vi "Evaluate Stop Trigger.vi"(8 "error in (no error)":errorcluster, 10 "Stop Trigger Data":dbl[](array[numeric]), 11 "Triggered Log in":refnum<class "Triggered Log.lvclass">) -> (0 "error out":errorcluster, 3 "Triggered Log out":refnum<class "Triggered Log.lvclass">)   [LabVIEW 2012, in "Triggered Log.lvclass"]
doc: "Evaluate the stop trigger if the log is in the Triggered state. Reset the posttrigger countdown so that when the stop trigger occurs it's ready. If the stop trigger occurs, set the log to the posttrigger state and notify any listeners of the state change."
uses:
  Triggered Log.lvclass
  Triggered Log.lvclass/Triggered Log.ctl
  Triggered Log State.ctl
  On Triggered Log State Change.vi
  Engine/Classes/Triggers/Trigger/Finalize.vi
  Engine/Classes/Triggers/Trigger/Trigger.lvclass
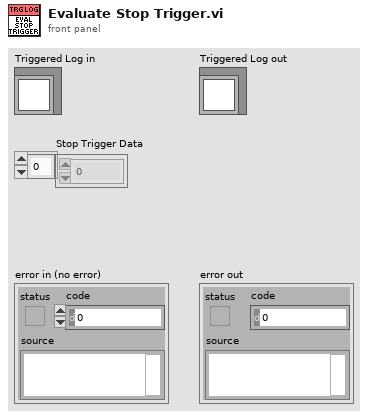
[diagram p1: front panel]
types:
  T1 = typedef "Triggered Log.lvclass/Triggered Log State.ctl" = enum16{"Waiting on Trigger", "Triggered", "Posttrigger", "Complete", "Idle", "Error"}
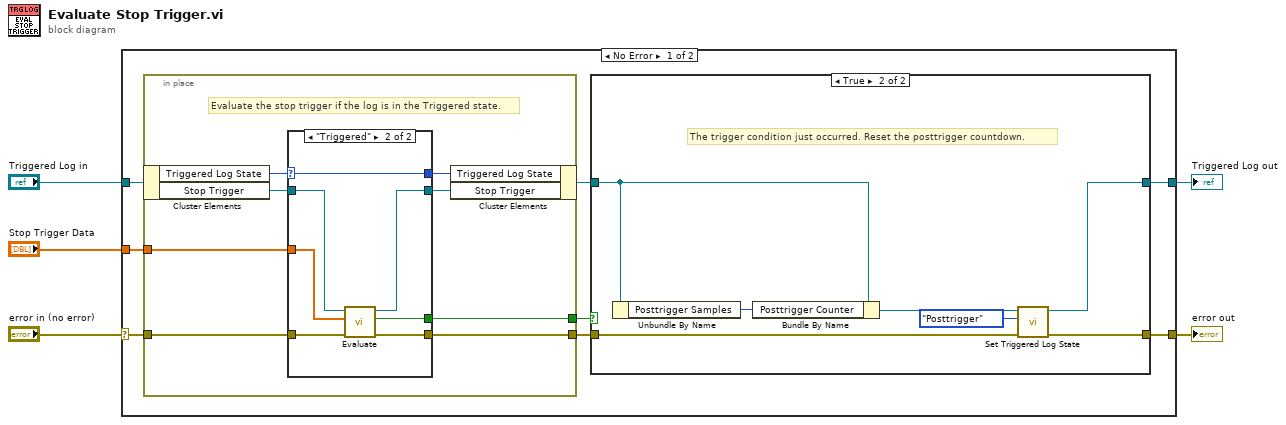
[diagram p0: block diagram]
diagram:
  n1 = case shown="No Error" "error in (no error)" {
    selector: "error in (no error)" -> [w6 w41]
    tunnel: "Stop Trigger Data" -> [w13 _]
    tunnel: "Triggered Log in" -> [w12 w42]
    tunnel: [w9 w41] -> w3
    tunnel: [w8 w42] -> w2
    frame No Error {
      n2 = in-place {
        in-place-border: w6 -> [w21]
        in-place-border: w13 -> [w19]
        in-place-border: [w20] -> w11
        in-place-border: [w16] -> w7
        # "Evaluate the stop trigger if the log is in the Triggered state."
        n3 = in-place-cluster #1(w12) -> ("Triggered Log State"=w17:T1, "Stop Trigger"=w15:refnum<class "Trigger.lvclass">)
        n4 = case shown="\"Triggered\"" w17 {
          selector: w17 -> [w24 w31]
          tunnel: w15 -> [w23 w30]
          tunnel: [w23 w26] -> w14
          tunnel: w21 -> [w22 w29]
          tunnel: [w22 w28] -> w20
          tunnel: w19 -> [_ w27]
          tunnel: [w24 w31] -> w18
          tunnel: [_ w25] -> w16
          frame Default {
            # "Only evaluate the trigger if the log is in theTriggered state."
          }
          frame "Triggered" {
            n5 = call "Evaluate.vi"("error in (no error)"=w29, "Trigger Data"=w27, "Trigger in"=w30) -> ("error out"=w28:errorcluster, "Trigger"=w25:bool, "Trigger out"=w26:refnum<class "Trigger.lvclass">)  [unwired: 6 in]
          }
        }
        n6 = in-place-cluster #1("Triggered Log State"=w18, "Stop Trigger"=w14) -> (w10:refnum<class "Triggered Log.lvclass">)
      }
      n7 = case shown="True" w7 {
        tunnel: w11 -> [w32 w38]
        tunnel: [w33 w39] -> w8
        tunnel: w10 -> [w33 w36]
        tunnel: [w32 w40] -> w9
        frame False {
        }
        frame True {
          # "The trigger condition just occurred. Reset the posttrigger countdown."
          n8 = Unbundle By Name(w36) -> ("Posttrigger Samples"=w34:i64)
          n9 = Bundle By Name(cluster=w36, "Posttrigger Counter"=w34) -> (w35:refnum<class "Triggered Log.lvclass">)
          n10 = call "Set Triggered Log State.vi"("error in (no error)"=w38, "Triggered Log State"=Triggered_Log_State."Posttrigger", "Triggered Log in"=w35) -> ("error out"=w40:errorcluster, "Triggered Log out"=w39:refnum<class "Triggered Log.lvclass">)  [unwired: 7 in]
        }
      }
    }
    frame Error {
    }
  }
  "error out" <- w3
  "Triggered Log out" <- w2
